vi "read_params.vi"(8 "error in (no error)":errorcluster, 11 "BernoulliNB in":refnum<class "BernoulliNB.lvclass">) -> (0 "error out":errorcluster, 2 "params":T1={"alpha"=1.0, "binarize"={"binarize_type"="float", "binarize_float"=0.0}, "fit_prior"=TRUE, "class_prior"={"class_prior_type"="None", "class_prior_list"=[]}}, 3 "BernoulliNB out":refnum<class "BernoulliNB.lvclass">)   [LabVIEW 2020, in "BernoulliNB.lvclass"]
uses:
  BernoulliNB.lvclass
  Controls/bernoulliNB_params.ctl
  BernoulliNB.lvclass/BernoulliNB.ctl
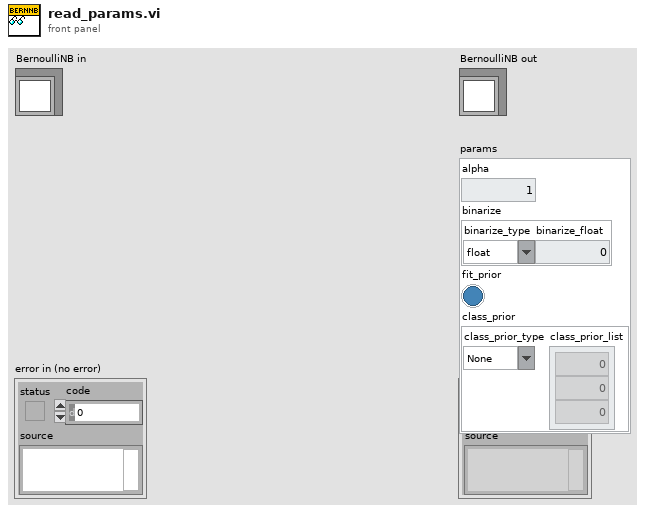
[diagram p1: front panel]
types:
  T1 = typedef "bernoulliNB_params.ctl" = cluster{"alpha":dbl, "binarize":cluster{"binarize_type":string, "binarize_float":dbl}, "fit_prior":bool, "class_prior":cluster{"class_prior_type":string, "class_prior_list":dbl[]}}
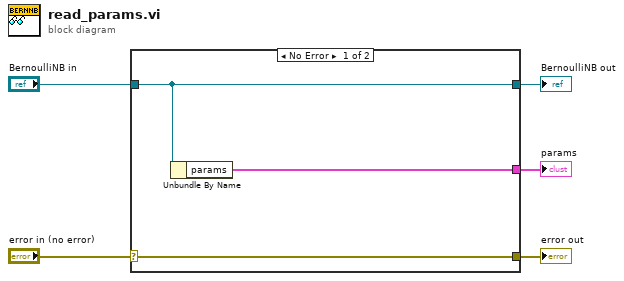
[diagram p0: block diagram]
diagram:
  n1 = case shown="No Error" "error in (no error)" {
    selector: "error in (no error)" -> [w8 w9]
    tunnel: [w8 w9] -> w4
    tunnel: [w7 w10] -> w2
    tunnel: "BernoulliNB in" -> [w7 w10]
    tunnel: [w6 _] -> w1
    frame No Error {
      n2 = Unbundle By Name(w7) -> ("params"=w6:T1)
    }
    frame Error {
    }
  }
  "error out" <- w4
  "BernoulliNB out" <- w2
  "params" <- w1
